vi "Remove Panel from SubPanel.vi"(8 "error in (no error)":errorcluster, 10 "Panel In":refnum<class "Panel.lvclass">, 11 "Manager in":refnum<class "Manager.lvclass">) -> (0 "error out":errorcluster, 2 "Panel":refnum<class "Panel.lvclass">, 3 "Manager out":refnum<class "Manager.lvclass">)   [LabVIEW 2020, in "OOPanel.lvlib" / "Manager.lvclass"]
uses:
  Manager.lvclass
  Panel/Panel.lvclass
  Panel/Visibility State.ctl
  OOPanel.lvlib
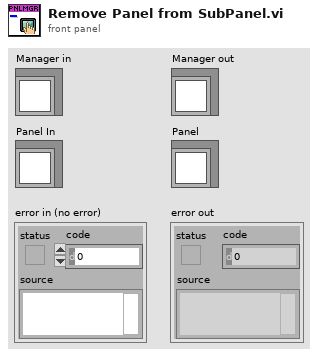
[diagram p1: front panel]
types:
  T1 = typedef "OOPanel.lvlib/Visibility State.ctl" = enum16{"Idle", "Closed", "Hidden", "Visible", "Subpanel"}
  T2 = typedef "OOPanel.lvlib/Manager.lvclass/Ref Data.ctl" = cluster{"SubPanel Map":T3, "Panels":refnum<class "Panel.lvclass">[]}
  T3 = typedef "OOPanel.lvlib/Manager.lvclass/SubPanel Map.ctl" = cluster{"SubPanels":refnum<vi>[], "Panels":refnum<class "Panel.lvclass">[]}
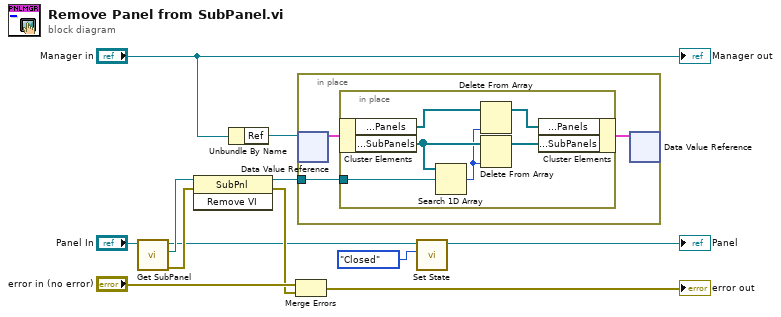
[diagram p0: block diagram]
diagram:
  n1 = call "Get SubPanel.vi"("Panel in"="Panel In") -> ("error out"=w7:errorcluster, "SubPanel"=w6:refnum<vi>, "Panel out"=w3:refnum<class "Panel.lvclass">)  [unwired: 8 in]
  n2 = invoke class="SubPnl" method="Remove VI"(reference=w6, error in=w7) -> (reference out=w8:refnum<vi>, error out=w4:errorcluster)  [unwired: 1 in, 1 out]
  n3 = Unbundle By Name("Manager in") -> ("Ref"=w10:refnum<data-value>)
  n4 = Merge Errors("error in (no error)", w4) -> (→"error out":errorcluster)
  n5 = in-place {
    in-place-border: w8 -> [w13]
    n6 = in-place-dvr #1(w10) -> (w15:T2)  [unwired: 1 out]
    n7 = in-place {
      in-place-border: w13 -> [w21]
      n8 = in-place-cluster #2(w15) -> ("SubPanel Map.Panels"=w18:refnum<class "Panel.lvclass">[], "SubPanel Map.SubPanels"=w20:refnum<vi>[])
      n9 = Search 1D Array(1D array=w20, element=w21) -> (index of element=w16:i32)  [unwired: 1 in]
      n10 = Delete From Array(array=w18, index=w16) -> (array with subset deleted=w17:refnum<class "Panel.lvclass">[])  [unwired: 1 in, 1 out]
      n11 = Delete From Array(array=w20, index=w16) -> (array with subset deleted=w19:refnum<vi>[])  [unwired: 1 in, 1 out]
      n12 = in-place-cluster #2("SubPanel Map.Panels"=w17, "SubPanel Map.SubPanels"=w19) -> (w14:T2)
    }
    n13 = in-place-dvr #1(w14) -> ()  [unwired: 2 out]
  }
  n14 = call "Set State.vi"("State"=Visibility_State."Closed", "Panel in"=w3) -> ("Panel out"=→"Panel":refnum<class "Panel.lvclass">)  [unwired: 8 in, 1 out]
  "Manager out" <- "Manager in"
